vi "Create index typedef.vi"(8 "error in (no error)":errorcluster) -> (0 "error out":errorcluster)   [LabVIEW 2016]
uses:
  <vilib>/Utility/miscctls.llb/LVPointTypeDef.ctl
  <vilib>/Utility/traverseref.llb/TRef TravTarget.ctl
  <vilib>/numeric/LVNumericRepresentation.ctl
  <vilib>/Utility/miscctls.llb/LVMinMaxIncTypeDef.ctl
  <vilib>/Utility/traverseref.llb/VI Scripting - Traverse.lvlib
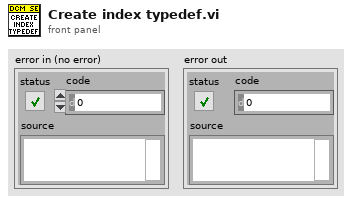
[diagram p1: front panel]
types:
  T1 = enum32{"invalid VI type", "Standard VI", "Control VI", "Global VI", "Polymorphic VI", "Configuration VI", "SubSystem", "Facade VI", "Method VI", "Statechart Diagram VI"}
  T2 = typedef "TRef TravTarget.ctl" = enum16{"FP", "BD", "Other"}
  T3 = typedef "LVPointTypeDef.ctl" = cluster{"Horizontal":i16, "Vertical":i16}
  T4 = enum32{"not a control VI", "control", "typedef", "strict typedef"}
  T5 = typedef "LVNumericRepresentation.ctl" = enum32{"Extended Precision", "Double Precision", "Single Precision", "Long", "Word", "Byte", "Unsigned Long", "Unsigned Word", "Unsigned Byte", "Complex Extended", "Complex Double", "Complex Single", "Quad", "Unsigned Quad", "Fixed-Point"}
  T6 = typedef "LVMinMaxIncTypeDef.ctl" = cluster{"Minimum":dbl, "Maximum":dbl, "Increment":dbl}
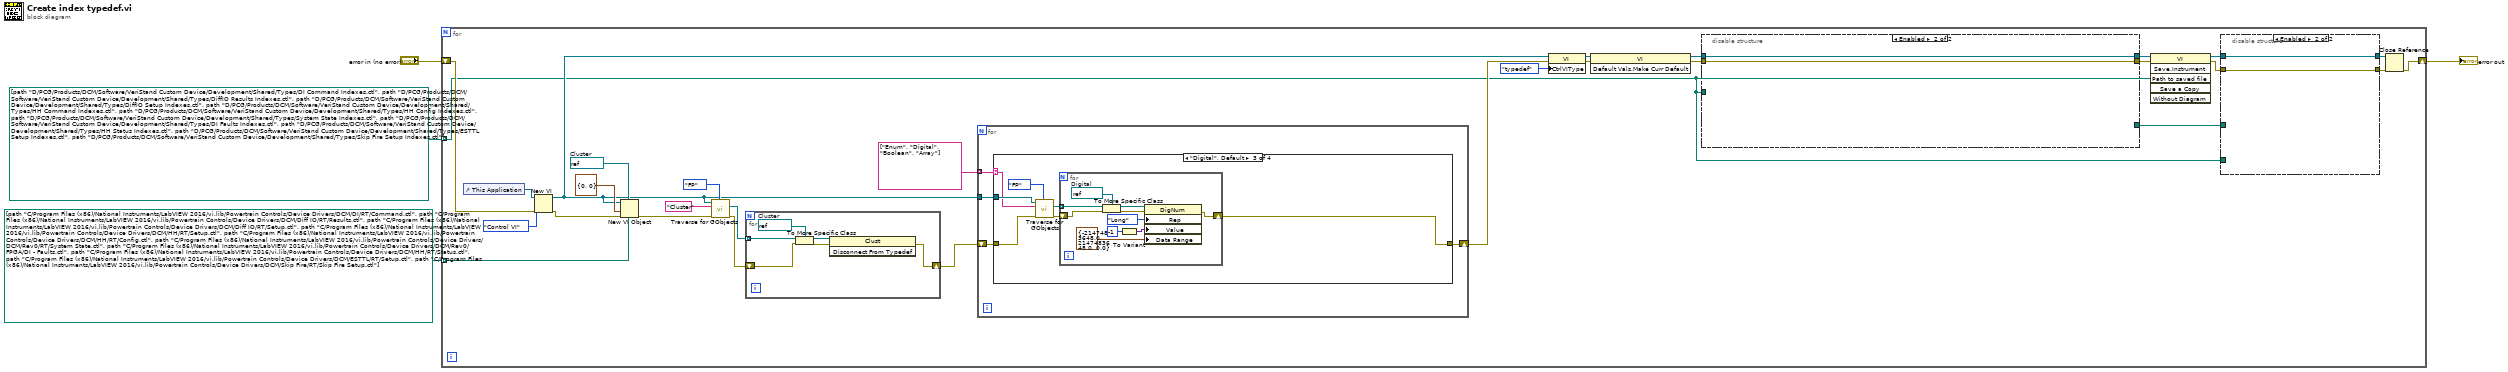
[diagram p0: block diagram]
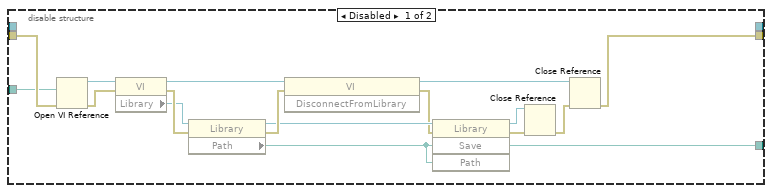
[diagram p2: hidden frame]
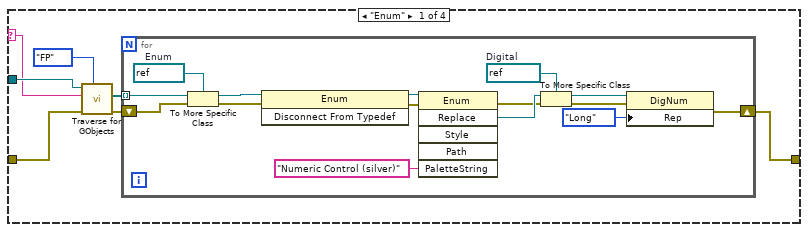
[diagram p3: hidden frame]
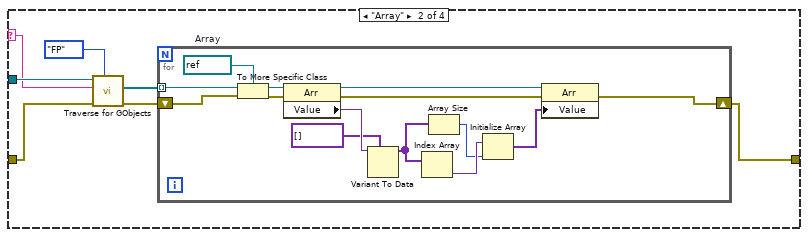
[diagram p4: hidden frame]
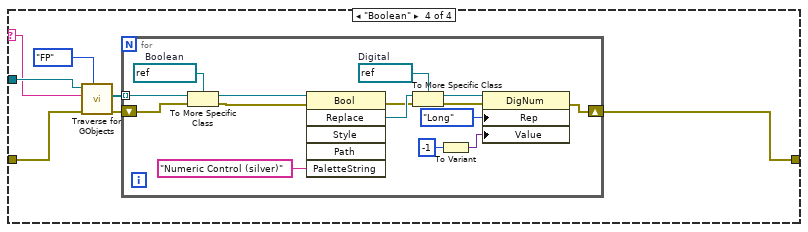
[diagram p5: hidden frame]
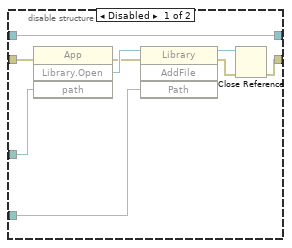
[diagram p6: hidden frame]
diagram:
  n1 = for {
    tunnel: path[] [path "D:/PCG/Products/DCM/Software/VeriStand Custom Device/Development/Shared/Types/DI Command Indexes.ctl", path "D:/PCG/Products/DCM/Software/VeriStand Custom Device/Development/Shared/Types/DiffIO Results Indexes.ctl", path "D:/PCG/Products/DCM/Software/VeriStand Custom Device/Development/Shared/Types/DiffIO Setup Indexes.ctl", path "D:/PCG/Products/DCM/Software/VeriStand Custom Device/Development/Shared/Types/HH Command Indexes.ctl", path "D:/PCG/Products/DCM/Software/VeriStand Custom Device/Development/Shared/Types/HH Config Indexes.ctl", path "D:/PCG/Products/DCM/Software/VeriStand Custom Device/Development/Shared/Types/System State Indexes.ctl", path "D:/PCG/Products/DCM/Software/VeriStand Custom Device/Development/Shared/Types/DI Faults Indexes.ctl", path "D:/PCG/Products/DCM/Software/VeriStand Custom Device/Development/Shared/Types/HH Status Indexes.ctl", path "D:/PCG/Products/DCM/Software/VeriStand Custom Device/Development/Shared/Types/ESTTL Setup Indexes.ctl", path "D:/PCG/Products/DCM/Software/VeriStand Custom Device/Development/Shared/Types/Skip Fire Setup Indexes.ctl"] -> [w9] mode=indexing
    tunnel: path[] [path "C:/Program Files (x86)/National Instruments/LabVIEW 2016/vi.lib/Powertrain Controls/Device Drivers/DCM/DI/RT/Command.ctl", path "C:/Program Files (x86)/National Instruments/LabVIEW 2016/vi.lib/Powertrain Controls/Device Drivers/DCM/Diff IO/RT/Results.ctl", path "C:/Program Files (x86)/National Instruments/LabVIEW 2016/vi.lib/Powertrain Controls/Device Drivers/DCM/Diff IO/RT/Setup.ctl", path "C:/Program Files (x86)/National Instruments/LabVIEW 2016/vi.lib/Powertrain Controls/Device Drivers/DCM/HH/RT/Setup.ctl", path "C:/Program Files (x86)/National Instruments/LabVIEW 2016/vi.lib/Powertrain Controls/Device Drivers/DCM/HH/RT/Config.ctl", path "C:/Program Files (x86)/National Instruments/LabVIEW 2016/vi.lib/Powertrain Controls/Device Drivers/DCM/Rev0/RT/System State.ctl", path "C:/Program Files (x86)/National Instruments/LabVIEW 2016/vi.lib/Powertrain Controls/Device Drivers/DCM/Rev0/FPGA/DI - Faults.ctl", path "C:/Program Files (x86)/National Instruments/LabVIEW 2016/vi.lib/Powertrain Controls/Device Drivers/DCM/HH/RT/Status.ctl", path "C:/Program Files (x86)/National Instruments/LabVIEW 2016/vi.lib/Powertrain Controls/Device Drivers/DCM/ESTTL/RT/Setup.ctl", path "C:/Program Files (x86)/National Instruments/LabVIEW 2016/vi.lib/Powertrain Controls/Device Drivers/DCM/Skip Fire/RT/Skip Fire Setup.ctl"] -> [w19] mode=indexing
    shift-right: [w17] -> w4
    shift-left: "error in (no error)" -> [w18]
    w33 = refnum<vi> refnum  # Cluster
    n2 = control-ref of="This Application"() -> (w21:refnum<vi>)
    n3 = New VI(8:w18, 9:T1."Control VI" ("vi type (standard vi)"), 11:w21) -> (0:w22:errorcluster, 3:w23:refnum<vi>)  [unwired: 4 in]
    n4 = New VI Object(vi object class=w33, owner refnum=w23, position/next to=T3 {"Horizontal"=0, "Vertical"=0} ("location"), 6:w19, 8:w22) -> (0:w30:errorcluster)  [unwired: 3 in, 1 out]
    n5 = call <vilib>:"Traverse for GObjects.vi"("Traverse Target"=TRef_TravTarget."FP", "error in (no error)"=w30, "Class Name"="Cluster", "VI Refnum"=w23) -> ("error out"=w29:errorcluster, "References"=w28:refnum<vi>[])  [unwired: 4 in, 2 out]
    n6 = for {
      shift-right: [w144] -> w27
      shift-left: w29 -> [w139]
      tunnel: w28 -> [w142] mode=indexing
      w143 = refnum<vi> refnum  # Cluster
      n7 = To More Specific Class(target class=w143, reference=w142, error in=w139) -> (specific class reference=w141:refnum<vi>, error out=w140:errorcluster)
      n8 = invoke class="Clust" method="Disconnect From Typedef"(reference=w141, error in=w140) -> (error out=w144:errorcluster)  [unwired: 1 in, 2 out]
    }
    n9 = for {
      tunnel: w23 -> [w55]
      shift-right: [w56] -> w24
      shift-left: w27 -> [w54]
      tunnel: string[] ["Enum", "Digital", "Boolean", "Array"] -> [w53] mode=indexing
      n10 = case shown="\"Digital\", Default" w53 {
        selector: w53 -> [w57 w83 w100 w117]
        tunnel: [w60 w79 w103 w120] -> w56
        tunnel: w55 -> [w59 w84 w102 w119]
        tunnel: w54 -> [w58 w82 w101 w118]
        frame "Enum" {
          n11 = call <vilib>:"Traverse for GObjects.vi"("Traverse Target"=TRef_TravTarget."FP", "error in (no error)"=w58, "Class Name"=w57, "VI Refnum"=w59) -> ("error out"=w62:errorcluster, "References"=w63:refnum<vi>[])  [unwired: 4 in, 2 out]
          n12 = for {
            tunnel: w63 -> [w78] mode=indexing
            shift-right: [w74] -> w60
            shift-left: w62 -> [w75]
            w69 = refnum<vi> refnum  # Digital
            w77 = refnum<vi> refnum  # Enum
            n13 = To More Specific Class(target class=w77, reference=w78, error in=w75) -> (specific class reference=w73:refnum<vi>, error out=w72:errorcluster)
            n14 = invoke class="Enum" method="Disconnect From Typedef"(reference=w73, error in=w72) -> (reference out=w71:refnum<vi>, error out=w70:errorcluster)  [unwired: 1 in, 1 out]
            n15 = invoke class="Enum" method="Replace"(reference=w71, error in=w70, "PaletteString"="Numeric Control (silver)" ("Palette String")) -> (error out=w65:errorcluster, "Replace"=w68:refnum<vi>)  [unwired: 3 in, 4 out]
            n16 = To More Specific Class(target class=w69, reference=w68, error in=w65) -> (specific class reference=w67:refnum<vi>, error out=w66:errorcluster)
            n17 = property class="DigNum"(reference=w67, error in=w66, "Rep"=LVNumericRepresentation."Long" ("Representation")) -> (error out=w74:errorcluster)  [unwired: 1 out]
          }
        }
        frame "Array" {
          n18 = call <vilib>:"Traverse for GObjects.vi"("Traverse Target"=TRef_TravTarget."FP", "error in (no error)"=w82, "Class Name"=w83, "VI Refnum"=w84) -> ("error out"=w80:errorcluster, "References"=w81:refnum<vi>[])  [unwired: 4 in, 2 out]
          n19 = for {
            tunnel: w81 -> [w98] mode=indexing
            shift-right: [w94] -> w79
            shift-left: w80 -> [w97]
            w99 = refnum<vi> refnum  # Array
            n20 = To More Specific Class(target class=w99, reference=w98, error in=w97) -> (specific class reference=w93:refnum<vi>, error out=w92:errorcluster)
            n21 = property class="Arr"(reference=w93, error in=w92) -> (reference out=w96:refnum<vi>, error out=w95:errorcluster, "Value"=w91:variant)
            n22 = Variant To Data(type=variant[] [], Variant=w91) -> (data=w87:variant[])  [unwired: 1 in, 1 out]
            n23 = Index Array(array=w87) -> (element=w89:variant)  [unwired: 1 in]
            n24 = Array Size(array=w87) -> (size(s)=w86:i32)
            n25 = Initialize Array(w89, w86) -> (w88:variant[])
            n26 = property class="Arr"(reference=w96, error in=w95, "Value"=w88) -> (error out=w94:errorcluster)  [unwired: 1 out]
          }
        }
        frame "Digital", Default {
          n27 = call <vilib>:"Traverse for GObjects.vi"("Traverse Target"=TRef_TravTarget."FP", "error in (no error)"=w101, "Class Name"=w100, "VI Refnum"=w102) -> ("error out"=w105:errorcluster, "References"=w106:refnum<vi>[])  [unwired: 4 in, 2 out]
          n28 = for {
            tunnel: w106 -> [w111] mode=indexing
            shift-right: [w115] -> w103
            shift-left: w105 -> [w110]
            w114 = refnum<vi> refnum  # Digital
            n29 = To More Specific Class(target class=w114, reference=w111, error in=w110) -> (specific class reference=w113:refnum<vi>, error out=w112:errorcluster)
            n30 = To Variant(anything=-1) -> (Variant=w108:variant)
            n31 = property class="DigNum"(reference=w113, error in=w112, "Rep"=LVNumericRepresentation."Long" ("Representation"), "Value"=w108, "Data Range"=T6 {"Minimum"=-2147483648.0, "Maximum"=2147483648.0, "Increment"=0.0} ("Data Entry Limits")) -> (error out=w115:errorcluster)  [unwired: 1 out]
          }
        }
        frame "Boolean" {
          n32 = call <vilib>:"Traverse for GObjects.vi"("Traverse Target"=TRef_TravTarget."FP", "error in (no error)"=w118, "Class Name"=w117, "VI Refnum"=w119) -> ("error out"=w122:errorcluster, "References"=w123:refnum<vi>[])  [unwired: 4 in, 2 out]
          n33 = for {
            tunnel: w123 -> [w138] mode=indexing
            shift-right: [w134] -> w120
            shift-left: w122 -> [w135]
            w133 = refnum<vi> refnum  # Digital
            w137 = refnum<vi> refnum  # Boolean
            n34 = To More Specific Class(target class=w137, reference=w138, error in=w135) -> (specific class reference=w128:refnum<vi>, error out=w127:errorcluster)
            n35 = invoke class="Bool" method="Replace"(reference=w128, error in=w127, "PaletteString"="Numeric Control (silver)" ("Palette String")) -> (error out=w129:errorcluster, "Replace"=w132:refnum<vi>)  [unwired: 3 in, 4 out]
            n36 = To More Specific Class(target class=w133, reference=w132, error in=w129) -> (specific class reference=w131:refnum<vi>, error out=w130:errorcluster)
            n37 = To Variant(anything=-1) -> (Variant=w124:variant)
            n38 = property class="DigNum"(reference=w131, error in=w130, "Rep"=LVNumericRepresentation."Long" ("Representation"), "Value"=w124) -> (error out=w134:errorcluster)  [unwired: 1 out]
          }
        }
      }
    }
    n39 = property class="VI"(reference=w23, error in=w24, "CtrlVIType"=T4."typedef" ("Control VI Type")) -> (reference out=w16:refnum<vi>, error out=w15:errorcluster)
    n40 = invoke class="VI" method="Default Vals.Make Curr Default"(reference=w16, error in=w15) -> (reference out=w8:refnum<vi>, error out=w13:errorcluster)  [unwired: 1 in, 1 out]
    n41 = disable-structure shown="Enabled" {
      disable-tunnel: [w46 w52] -> w14
      disable-tunnel: w13 -> [w49 w52]
      disable-tunnel: w9 -> [w47 _]
      disable-tunnel: [w39 _] -> w10
      disable-tunnel: w8 -> [_ w51]
      disable-tunnel: [_ w51] -> w7
      frame Disabled {
        n42 = Open VI Reference(vi path=w47, error in (no error)=w49) -> (vi reference=w50:refnum<vi>, error out=w48:errorcluster)  [unwired: 4 in]
        n43 = property class="VI"(reference=w50, error in=w48) -> (reference out=w45:refnum<vi>, error out=w43:errorcluster, "Library"=w42:refnum<vi>)
        n44 = property class="Library"(reference=w42, error in=w43) -> (reference out=w37:refnum<vi>, error out=w41:errorcluster, "Path"=w39:path)
        n45 = invoke class="VI" method="DisconnectFromLibrary"(reference=w45, error in=w41) -> (reference out=w44:refnum<vi>, error out=w36:errorcluster)  [unwired: 1 in, 1 out]
        n46 = invoke class="Library" method="Save"(reference=w37, error in=w36, "Path"=w39) -> (reference out=w38:refnum<vi>, error out=w35:errorcluster)  [unwired: 1 in, 2 out]
        n47 = Close Reference(reference=w38, error in (no error)=w35) -> (error out=w40:errorcluster)
        n48 = Close Reference(reference=w44, error in (no error)=w40) -> (error out=w46:errorcluster)
      }
      frame Enabled {
      }
    }
    n49 = invoke class="VI" method="Save.Instrument"(reference=w7, error in=w14, "Path to saved file"=w9) -> (reference out=w5:refnum<vi>, error out=w11:errorcluster)  [unwired: 3 in, 4 out]
    n50 = disable-structure shown="Enabled" {
      disable-tunnel: [w151 w155] -> w12
      disable-tunnel: w11 -> [w150 w155]
      disable-tunnel: w10 -> [w149 _]
      disable-tunnel: w9 -> [w146 _]
      disable-tunnel: [w145 w154] -> w6
      disable-tunnel: w5 -> [w145 w154]
      frame Disabled {
        n51 = invoke class="App" method="Library.Open"(error in=w150, "path"=w149) -> (error out=w147:errorcluster, "Open Library"=w148:refnum<vi>)  [unwired: 2 in, 2 out]
        n52 = invoke class="Library" method="AddFile"(reference=w148, error in=w147, "Path"=w146) -> (reference out=w152:refnum<vi>, error out=w153:errorcluster)  [unwired: 1 in, 2 out]
        n53 = Close Reference(reference=w152, error in (no error)=w153) -> (error out=w151:errorcluster)
      }
      frame Enabled {
      }
    }
    n54 = Close Reference(reference=w6, error in (no error)=w12) -> (error out=w17:errorcluster)
  }
  "error out" <- w4
